vi "TestMetronome.vi"() -> ()   [LabVIEW 2020]
panel:
  in  "Timing (ms)":i32(slide) scale=100.0..1000.0
  in  "Error Button":bool
  out "LED":bool
  in  "Stop Button":bool
  in  "Pause Button":bool
  in  "Start Button":bool
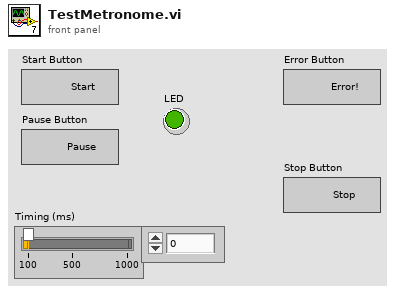
[diagram p1: front panel]
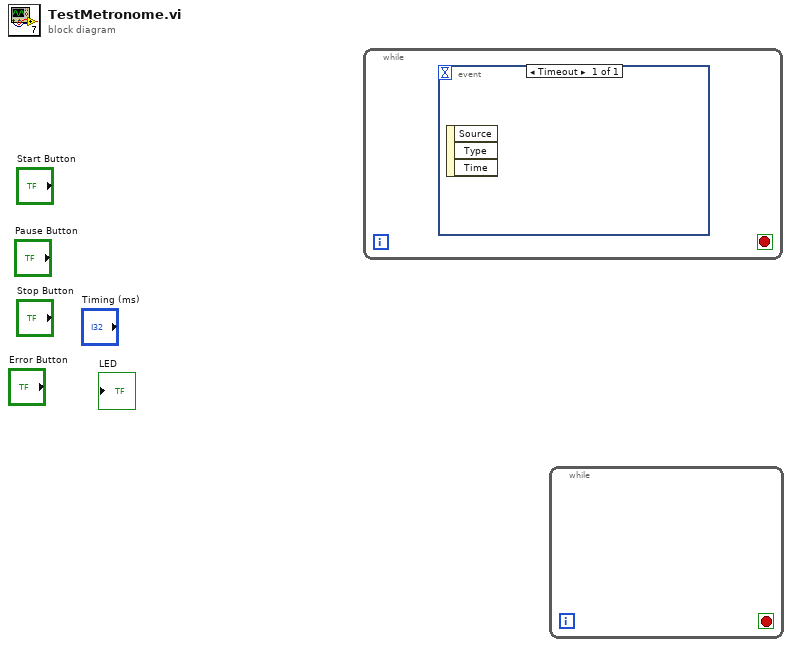
[diagram p0: block diagram]
diagram:
  n1 = while {
    stop <- _ stop-if-true
    n2 = event shown="[0] Timeout" {
      selector: _ -> [_]
      dyn-events: _ -> [_]
      timeout: _ -> [_]
      event Timeout {
        n3 = event-data() -> ()  [unwired: 1 in, 3 out]
      }
    }
  }
  n4 = while {
    stop <- _ stop-if-true
  }
